vi "program_pulse_blaster.vi"(7 "Sync Experiment":bool, 8 "error in (no error)":errorcluster, 9 "Instructions":T2(array[cluster]), 11 "Ramp Delay Settings":T1={"Subroutine A"=[{"Instruct Data"=6, "Op Code"=0, "Flags"=[TRUE, FALSE, FALSE, FALSE, TRUE, TRUE, FALSE, TRUE, FALSE, TRUE, FALSE, FALSE, FALSE, FALSE, FALSE, FALSE, TRUE, TRUE, FALSE, FALSE, FALSE, FALSE, TRUE, FALSE], "Comments"="Blue MOT", "Time (s)"=2.0}, {"Instruct Data"=9, "Op Code"=0, "Flags"=[TRUE, FALSE, FALSE, FALSE, FALSE, TRUE, FALSE, TRUE, FALSE, TRUE, FALSE, FALSE, TRUE, FALSE, FALSE, FALSE, TRUE, TRUE, FALSE, FALSE, FALSE, FALSE, TRUE, FALSE], "Comments"="Hold", "Time (s)"=0.1}, {"Instruct Data"=11, "Op Code"=0, "Flags"=[TRUE, FALSE, FALSE, FALSE, FALSE, FALSE, FALSE, TRUE, FALSE, TRUE, FALSE, FALSE, TRUE, FALSE, FALSE, FALSE, TRUE, TRUE, FALSE, FALSE, FALSE, FALSE, TRUE, FALSE], "Comments"="Repump", "Time (s)"=0.05}, {"Instruct Data"=10, "Op Code"=0, "Flags"=[FALSE, FALSE, FALSE, FALSE, FALSE, TRUE, TRUE, FALSE, TRUE, FALSE, FALSE, TRUE, TRUE, FALSE, FALSE, FALSE, TRUE, FALSE, FALSE, FALSE, FALSE, FALSE, TRUE, FALSE], "Comments"="Red MOT", "Time (s)"=0.2}, {"Instruct Data"=11, "Op Code"=0, "Flags"=[FALSE, FALSE, FALSE, FALSE, FALSE, TRUE, TRUE, FALSE, TRUE, FALSE, FALSE, TRUE, TRUE, FALSE, FALSE, FALSE, FALSE, FALSE, FALSE, FALSE, FALSE, FALSE, TRUE, FALSE], "Comments"="Load ODT", "Time (s)"=0.1}, {"Instruct Data"=11, "Op Code"=0, "Flags"=[FALSE, FALSE, FALSE, FALSE, FALSE, TRUE, TRUE, TRUE, FALSE, FALSE, FALSE, TRUE, TRUE, FALSE, FALSE, FALSE, FALSE, FALSE, FALSE, FALSE, FALSE, FALSE, TRUE, FALSE], "Comments"="ODT Hold", "Time (s)"=0.5}, {"Instruct Data"=11, "Op Code"=0, "Flags"=[FALSE, FALSE, FALSE, FALSE, FALSE, TRUE, TRUE, TRUE, FALSE, FALSE, FALSE, TRUE, TRUE, FALSE, TRUE, FALSE, FALSE, FALSE, FALSE, FALSE, FALSE, FALSE, TRUE, FALSE], "Comments"="", "Time (s)"=0.8}, {"Instruct Data"=200, "Op Code"=2, "Flags"=[FALSE, FALSE, FALSE, FALSE, FALSE, TRUE, TRUE, TRUE, FALSE, FALSE, FALSE, TRUE, TRUE, TRUE, TRUE, FALSE, FALSE, FALSE, FALSE, FALSE, FALSE, TRUE, TRUE, FALSE], "Comments"="loop hold", "Time (s)"=0.01}, {"Instruct Data"=0, "Op Code"=0, "Flags"=[FALSE, FALSE, FALSE, FALSE, FALSE, TRUE, TRUE, TRUE, FALSE, FALSE, FALSE, TRUE, TRUE, TRUE, TRUE, FALSE, FALSE, FALSE, FALSE, FALSE, FALSE, TRUE, TRUE, TRUE], "Comments"="", "Time (s)"=2.5e-06}, {"Instruct Data"=0, "Op Code"=0, "Flags"=[FALSE, FALSE, FALSE, FALSE, FALSE, TRUE, TRUE, TRUE, FALSE, FALSE, FALSE, TRUE, TRUE, TRUE, TRUE, FALSE, FALSE, FALSE, FALSE, FALSE, FALSE, TRUE, TRUE, FALSE], "Comments"="expose uv", "Time (s)"=2e-06}, {"Instruct Data"=7, "Op Code"=3, "Flags"=[FALSE, FALSE, FALSE, FALSE, FALSE, TRUE, TRUE, TRUE, FALSE, FALSE, FALSE, TRUE, TRUE, TRUE, TRUE, FALSE, FALSE, FALSE, FALSE, FALSE, FALSE, TRUE, FALSE, FALSE], "Comments"="", "Time (s)"=1.5e-05}, {"Instruct Data"=0, "Op Code"=0, "Flags"=[FALSE, FALSE, FALSE, FALSE, FALSE, TRUE, TRUE, TRUE, FALSE, FALSE, FALSE, TRUE, TRUE, FALSE, FALSE, FALSE, TRUE, FALSE, FALSE, FALSE, FALSE, TRUE, TRUE, FALSE], "Comments"="Drop", "Time (s)"=0.01}, {"Instruct Data"=0, "Op Code"=0, "Flags"=[FALSE, TRUE, TRUE, TRUE, FALSE, TRUE, TRUE, TRUE, FALSE, FALSE, FALSE, TRUE, TRUE, FALSE, FALSE, FALSE, TRUE, FALSE, FALSE, FALSE, FALSE, FALSE, TRUE, FALSE], "Comments"="Image atoms ", "Time (s)"=1e-05}, {"Instruct Data"=0, "Op Code"=0, "Flags"=[FALSE, FALSE, TRUE, FALSE, FALSE, TRUE, TRUE, TRUE, FALSE, FALSE, FALSE, TRUE, TRUE, FALSE, FALSE, FALSE, TRUE, FALSE, FALSE, FALSE, FALSE, FALSE, TRUE, FALSE], "Comments"="Wait", "Time (s)"=0.081}, {"Instruct Data"=0, "Op Code"=0, "Flags"=[FALSE, TRUE, TRUE, TRUE, FALSE, TRUE, TRUE, TRUE, FALSE, FALSE, FALSE, TRUE, TRUE, FALSE, FALSE, FALSE, TRUE, FALSE, FALSE, FALSE, FALSE, FALSE, TRUE, FALSE], "Comments"="Image BG", "Time (s)"=1e-05}, {"Instruct Data"=0, "Op Code"=6, "Flags"=[FALSE, FALSE, FALSE, FALSE, FALSE, TRUE, TRUE, TRUE, FALSE, FALSE, FALSE, FALSE, TRUE, FALSE, FALSE, FALSE, TRUE, FALSE, FALSE, FALSE, FALSE, FALSE, TRUE, FALSE], "Comments"="Kill time", "Time (s)"=0.5}], "Insert Delays"=FALSE, "Number of loops"=0, "Insert after instruction"=0, "Random"=FALSE, "Initial Delay Time (s)"=0.0, "Final Delay Time (s)"=5e-08, "Delay Step (s)"=5e-08, "Delay Column"=0.0, "Loop Hold Column"=0.0, "Field Ramp Column"=0.0, "Excitation Column"=0.0, "Hold + Delay + Excitation Time"=0.0, "Ascending/Descending"=FALSE} {"Insert after instruction" min=0; "Delay Step (s)" min=5e-08 format="%#_6p"; "Final Delay Time (s)" min=5e-08 format="%#_6p"; "Initial Delay Time (s)" min=5e-08 format="%#_6p"; "Subroutine A"."Time (s)" min=5e-08 format="%.3p"; "Subroutine A"."Op Code" items=["Continue", "Stop", "Loop", "End Loop", "JSR", "RTS", "Branch", "Long Delay", "Wait"]; "Subroutine A"."Instruct Data" format="%.0p"}) -> (0 "error out":errorcluster, 3 "Tau Array Out":dbl[](array[numeric]))   [LabVIEW 2015]
uses:
  Controls/PulseBlaster/delay_control_2..ctl
panel:
  out "Numeric":i32
  # "1"
  # "2"
  # "3"
  # "4"
  # "5"
  # "6"
  # "7"
  # "8"
  # "9"
  # "10"
  # "11"
  # "12"
  # "13"
  # "14"
  # "15"
  # "16"
  # "17"
  # "18"
  # "19"
  # "20"
  # "21"
  # "22"
  # "23"
  # "24"
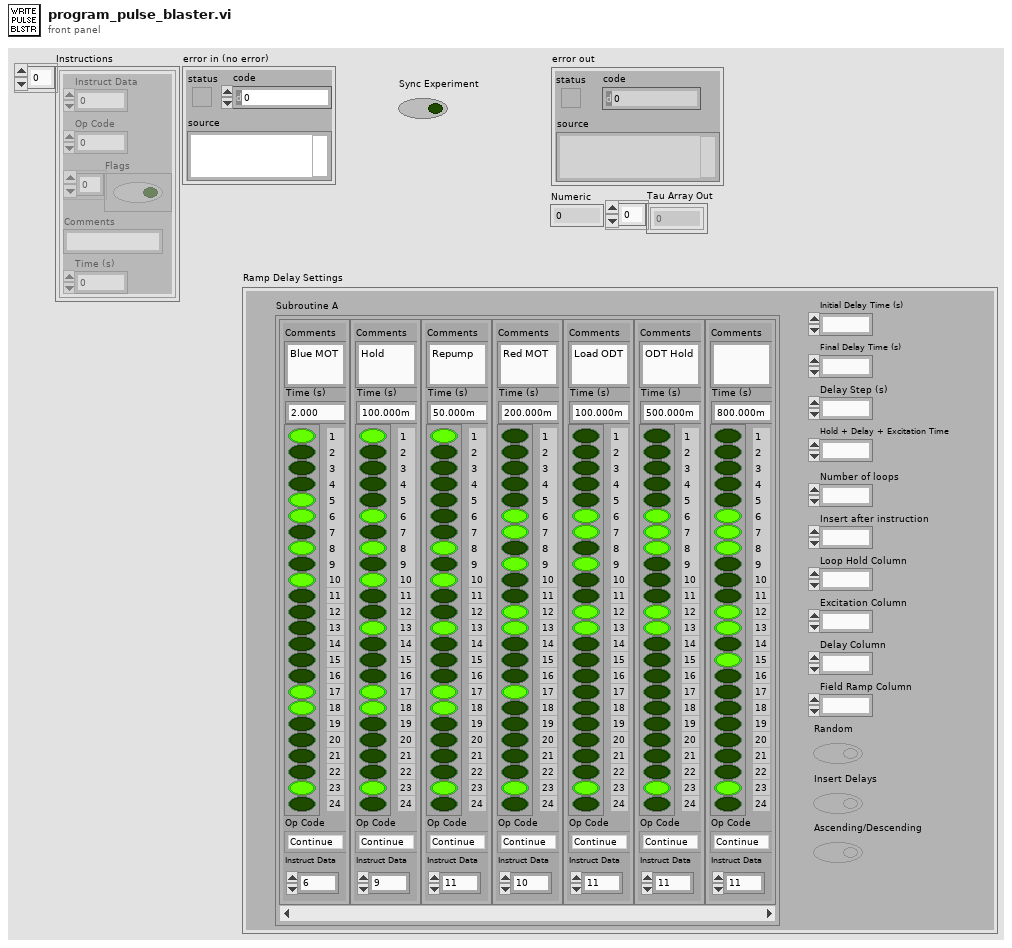
[diagram p1: front panel]
types:
  T1 = typedef "delay_control_2..ctl" = cluster{"Subroutine A":cluster{"Instruct Data":i32, "Op Code":i32, "Flags":bool[], "Comments":string, "Time (s)":dbl}[], "Insert Delays":bool, "Number of loops":i32, "Insert after instruction":i32, "Random":bool, "Initial Delay Time (s)":dbl, "Final Delay Time (s)":dbl, "Delay Step (s)":dbl, "Delay Column":dbl, "Loop Hold Column":dbl, "Field Ramp Column":dbl, "Excitation Column":dbl, "Hold + Delay + Excitation Time":dbl, "Ascending/Descending":bool}
  T2 = cluster{"Instruct Data":i32, "Op Code":i32, "Flags":bool[], "Comments":string, "Time (s)":dbl}[]
  T3 = enum16{"Pulse Program", "Frequency Registers", "TX Phase Registers", "RX Phase Registers"}
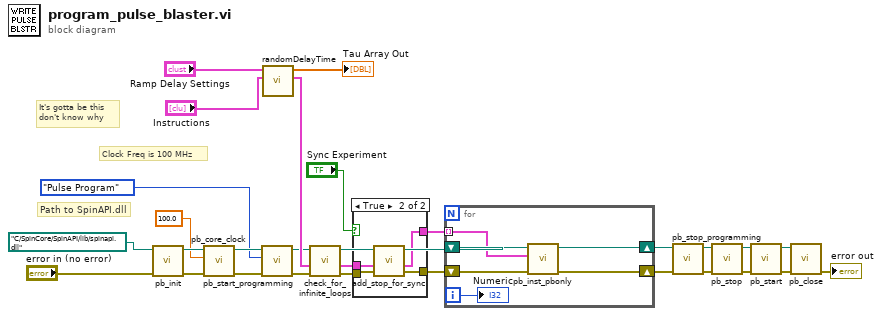
[diagram p0: block diagram]
diagram:
  # "It's gotta be this\ndon't know why"
  # "Clock Freq is 100 MHz"
  # "Path to SpinAPI.dll"
  n1 = call "pb_init.vi"("error in (no error)"="error in (no error)", "path in"=path "C:/SpinCore/SpinAPI/lib/spinapi.dll") -> ("error out"=w27:errorcluster, "path out"=w26:path)  [unwired: 2 in, 6 out]
  n2 = call "pb_core_clock.vi"("error in (no error)"=w27, "clock_freq (MHz)"=100.0, "path in"=w26) -> ("error out"=w24:errorcluster, "path out"=w23:path)  [unwired: 7 in]
  n3 = call "pb_start_programming.vi"("error in (no error)"=w24, "Device"=T3."Pulse Program", "path in"=w23) -> ("error out"=w12:errorcluster, "path out"=w6:path)  [unwired: 1 in, 6 out]
  n4 = call "randomDelayTime.vi"("Instructions"="Instructions", "Ramp Delay Settings"="Ramp Delay Settings") -> ("Instructions Out"=w11:T2, "Tau Array Out"=→"Tau Array Out":dbl[])  [unwired: 8 in]
  n5 = call "check_for_infinite_loops.vi"("error in (no error)"=w12, "Instructions"=w11) -> ("error out"=w7:errorcluster, "Instructions Out"=w10:T2)  [unwired: 8 in]
  n6 = case shown="True" "Sync Experiment" {
    tunnel: w10 -> [w29 w32]
    tunnel: [w29 w31] -> w9
    tunnel: [w30 w33] -> w8
    tunnel: w7 -> [w30 w33]
    frame False {
    }
    frame True {
      n7 = call "add_stop_for_sync.vi"("Instructions Out"=w32) -> ("Instructions Out 2"=w31:T2)  [unwired: 10 in]
    }
  }
  n8 = for {
    tunnel: w9 -> [w36] mode=indexing
    shift-right: [w38] -> w20
    shift-left: w6 -> [w39]
    shift-right: [w35] -> w21
    shift-left: w8 -> [w37]
    i -> [w34]
    n9 = call "pb_inst_pbonly.vi"("error in (no error)"=w37, "PB Instruction"=w36, "path in"=w39) -> ("error out"=w35:errorcluster, "path out"=w38:path)  [unwired: 2 in, 5 out]
    "Numeric" <- w34
  }
  n10 = call "pb_stop_programming.vi"("error in (no error)"=w21, "path in"=w20) -> ("error out"=w2:errorcluster, "path out"=w5:path)  [unwired: 1 in, 7 out]
  n11 = call "pb_stop.vi"("error in (no error)"=w2, "path in"=w5) -> ("error out"=w3:errorcluster, "path out"=w4:path)  [unwired: 8 in]
  n12 = call "pb_start.vi"("error in (no error)"=w3, "path in"=w4) -> ("error out"=w18:errorcluster, "path out"=w17:path)  [unwired: 8 in]
  n13 = call "pb_close.vi"("error in (no error)"=w18, "path in"=w17) -> ("error out"=→"error out":errorcluster)  [unwired: 9 out]
